vi "Junk test ping with dotNET.vi"() -> ()   [LabVIEW 2013]
panel:
  out "Ping output 2":string="\r\nPinging www.google.com [172.217.8.100] with 32 bytes of data:\r\nReply from 172.217.8.100: bytes=32 time=15ms TTL=56\r\nReply from 172.217.8.100: bytes=32 time=16ms TTL=56\r\nReply from 172.217.8.100: bytes=32 time=16ms TTL=56\r\nReply from 172.217.8.100: bytes=32 time=17ms TTL=56\r\n\r\nPing statistics for 172.217.8.100:\r\n    Packets: Sent = 4, Received = 4, Lost = 0 (0% loss),\r\nApproximate round trip times in milli-seconds:\r\n    Minimum = 15ms, Maximum = 17ms, Average = 16ms\r\n"
  out "error out":errorcluster
  out "Ping output":string
  in  "Ping options":string="www.google.com"
  in  "IP Address":string="www.google.com"
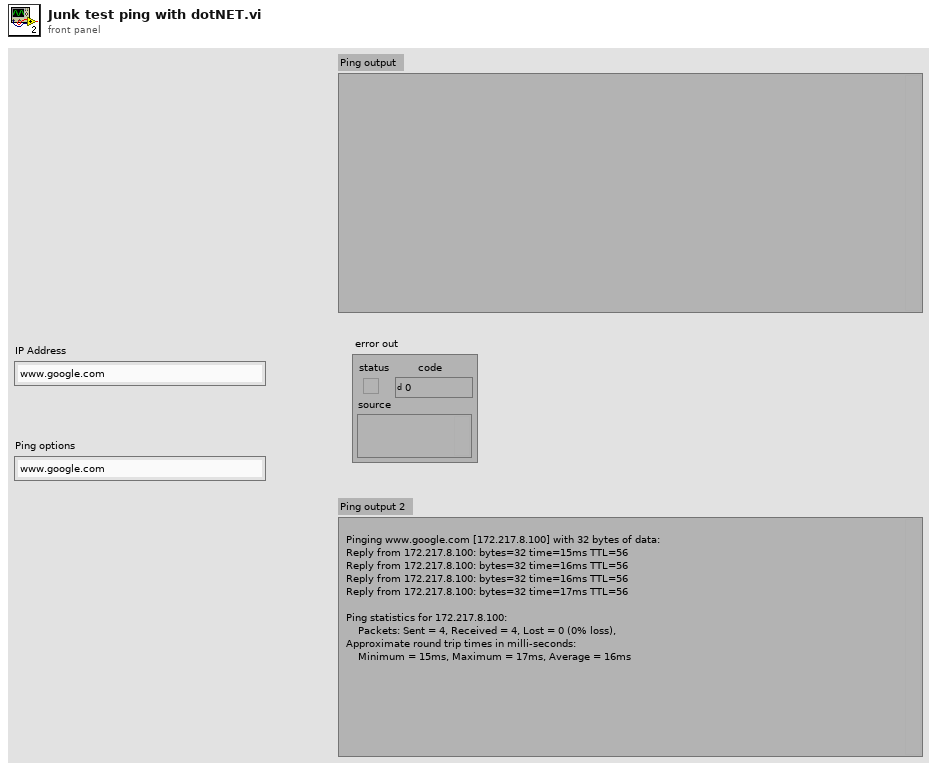
[diagram p1: front panel]
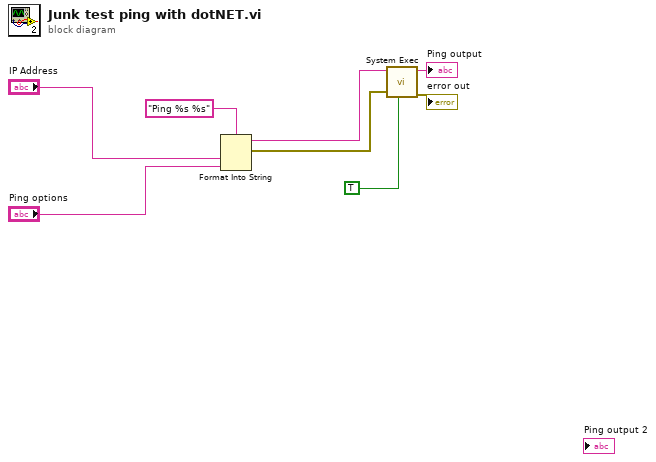
[diagram p0: block diagram]
diagram:
  n1 = Format Into String(format string="Ping %s %s", "IP Address", "Ping options") -> (resulting string=w5:string, error out=w3:errorcluster)  [unwired: 2 in]
  n2 = call <vilib>:"System Exec.vi"("run minimized? (F)"=TRUE, "error in (no error)"=w3, "command line"=w5) -> ("error out"=→"error out":errorcluster, "standard output"=→"Ping output":string)  [unwired: 5 in, 2 out]
